vi "1_03.vi"() -> ()   [LabVIEW 2013]
panel:
  out "Salida 2 [dB]":dbl
  in  "Entrada 2 [V]":dbl
  out "Salida [dB]":dbl
  in  "Entrada [V]":dbl
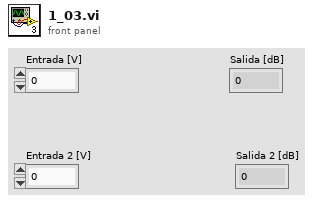
[diagram p1: front panel]
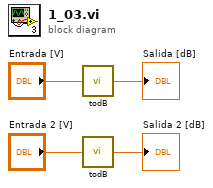
[diagram p0: block diagram]
diagram:
  n1 = call "todB.vi"("Entrada [V]"="Entrada [V]") -> ("Salida [dB]"=→"Salida [dB]":dbl)
  n2 = call "todB.vi"("Entrada [V]"="Entrada 2 [V]") -> ("Salida [dB]"=→"Salida 2 [dB]":dbl)
